vi "Orbit (SubVI).vi"(6 "error in (no error)":errorcluster, 9 "Axis Y1":tag="cDAQ1Mod1/ai1", 10 "Axis X1":tag="cDAQ1Mod1/ai0", 11 "Array":waveform(dbl)[](array[waveform])) -> (3 "Cluster":cluster{"Y":dbl[], "Y":dbl[]}, 8 "error out":errorcluster)   [LabVIEW 2012]
uses:
  <vilib>/Waveform/WDTOps.llb/WDT Index Channel by Name DBL.vi
  <vilib>/Analysis/baseanly.llb/Mean (DBL).vi
  <vilib>/Analysis/NI_AALBase.lvlib
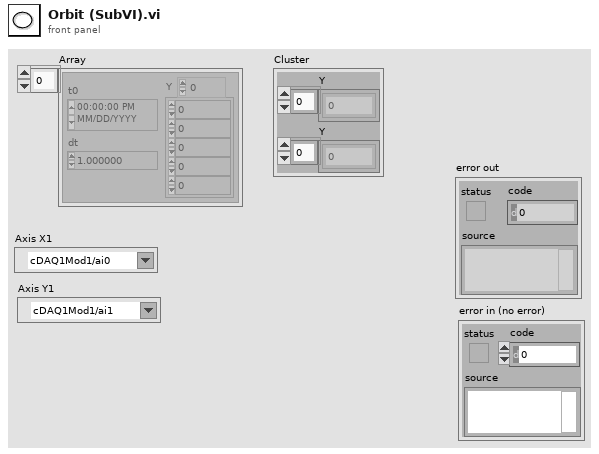
[diagram p1: front panel]
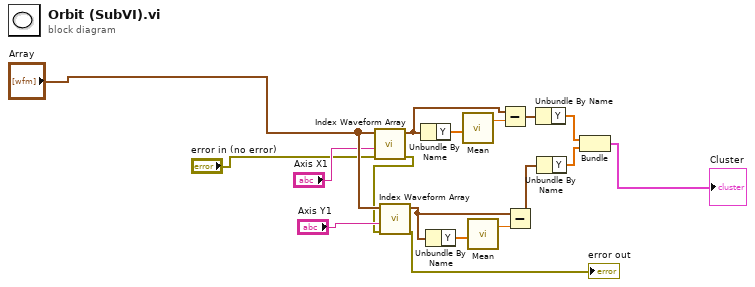
[diagram p0: block diagram]
diagram:
  n1 = call-poly <vilib>:"Index Waveform Array.vi"("error in (no error)"="error in (no error)", "channel name"="Axis X1", "waveform array"="Array") -> ("error out"=w3:errorcluster, "waveform"=w11:waveform(dbl))  [unwired: 7 in]
  n2 = call-poly <vilib>:"Index Waveform Array.vi"("error in (no error)"=w3, "channel name"="Axis Y1", "waveform array"="Array") -> ("error out"=→"error out":errorcluster, "waveform"=w7:waveform(dbl))  [unwired: 7 in]
  n3 = Unbundle By Name(w11) -> ("Y"=w10:dbl[])
  n4 = Unbundle By Name(w7) -> ("Y"=w6:dbl[])
  n5 = call-poly <vilib>:"Mean.vi"("X"=w10) -> ("mean"=w9:dbl)  [unwired: 1 out]
  n6 = call-poly <vilib>:"Mean.vi"("X"=w6) -> ("mean"=w8:dbl)  [unwired: 1 out]
  n7 = Subtract(x=w11, y=w9) -> (x-y=w15:waveform(dbl))
  n8 = Subtract(x=w7, y=w8) -> (x-y=w16:waveform(dbl))
  n9 = Unbundle By Name(w15) -> ("Y"=w12:dbl[])
  n10 = Unbundle By Name(w16) -> ("Y"=w13:dbl[])
  n11 = Bundle "Bundle"("Y"=w12, "Y"=w13) -> (→"Cluster":cluster{"Y":dbl[], "Y":dbl[]})  [unwired: 1 in]
